vi "Journal.vi"(11 "Journal Queue":refnum<queue>) -> ()   [LabVIEW 2013, in "main.lvlib"]
uses:
  main.lvlib
  Components/Dependencies.llb/amc_Message Queue.ctl
  Components/Dependencies.llb/amc_Message.ctl
  <vilib>/FTP/util/Keyed Array.ctl
  Controls/Enum Variables.ctl
  Controls/Reference AE Control.ctl
  Components/Dependencies.llb/TLB_Dependencies.lvlib
  <vilib>/FTP/NI_FTP.lvlib
panel:
  in  "Send To PACS":bool
  in  "Stop":bool
  in  "ReportSelection":u16(ring) caption="Journal" items=["Distal Tryk", "Hudperfusionstryk", "Distal Tryk: Finger", "Arbejdstest", "Finger stimulering"]
  in  "GenerateReport":bool
  in  "Data Menu":string(tree) caption="TreeMenu"
  in  "Data Listbox":i32(listbox)=-1
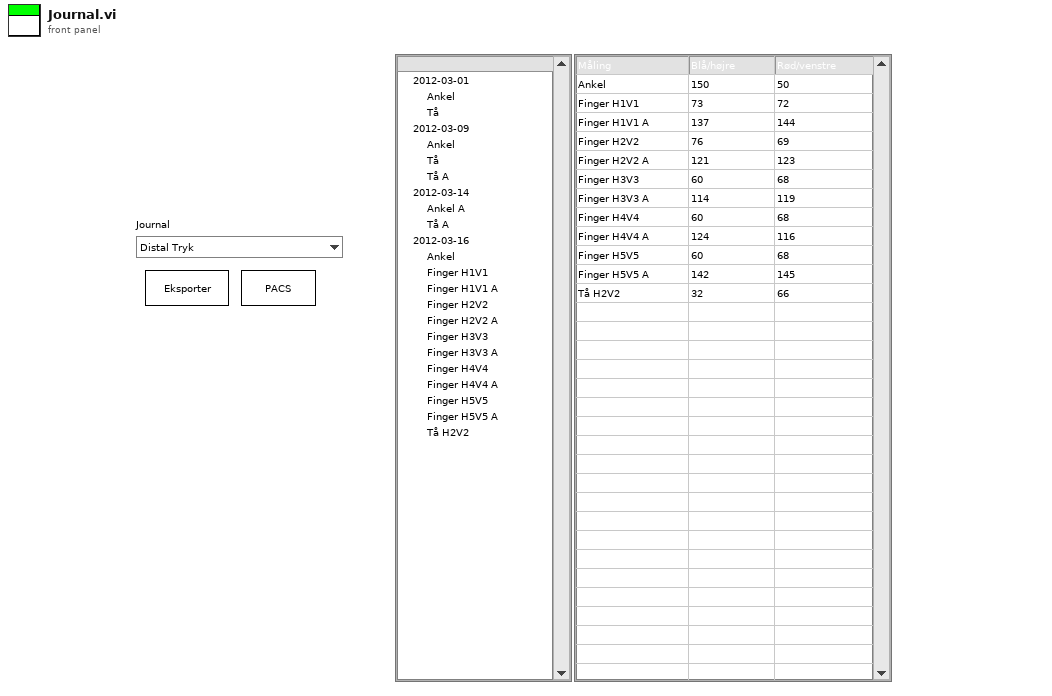
[diagram p1: front panel]
types:
  T1 = typedef "main.lvlib/TLB_Dependencies.lvlib/amc_Message Queue.ctl" = refnum<queue>
  T2 = typedef "main.lvlib/Reference AE Control.ctl" = enum16{"Initialize", "Set Menu", "Set Profile", "Set Configuration", "Set Configuration_old", "Set Configuration_new", "Set Configuration Method", "Set Acquisition", "Set Data", "Set Journal", "Get"}
  T3 = cluster{"ReportSelection":refnum<vi>, "Data Listbox":refnum<vi>, "GenerateReport":refnum<vi>, "Data Menu":refnum<vi>, "Send To PACS":refnum<vi>}
  T4 = typedef "main.lvlib/Enum Variables.ctl" = enum16{"SetAcqFilter", "GetAcqFilter", "Set Filter", "Get Filter", "Set Height", "Get Height", "Set Recorded Height", "Get Recorded Height", "Set Blue Pressure", "Get Blue Pressure", "Set Red Pressure", "Get Red Pressure", "Init", "Reset Pressure", "Set Red Cursors", "Get Red Cursors", "Set Blue Cursors", "Get Blue Cursors", "Set Language", "Get Language", "Set Active Graphs", "Get ActiveGraphs", "Set Method", "Get Method", "Set Encryption", "Get Encryption", "Set ExcelVersion", "Get ExcelVersion", "Set DICOM Avail", "Get DICOM Avail", "Set DICOM Encode", "Get DICOM Encode", "Set JournalExport", "Get JournalExport", "Set Sequence", "Get Sequence", "Set DAQ Connected", "Get DAQ Connected", "Set Current Graph", "Get Current Graph", "Set General Settings", "Get Hyphenation", "Set Arm Calc Method", "Get Arm Calc Method", "Set Dicom Tags", "Get Dicom Tags", "Set BT Serial", "Get BT Serial", "Set BT Accepted Serials", "Get BT Accepted Serials", "Get BT License", "Set BT License"}
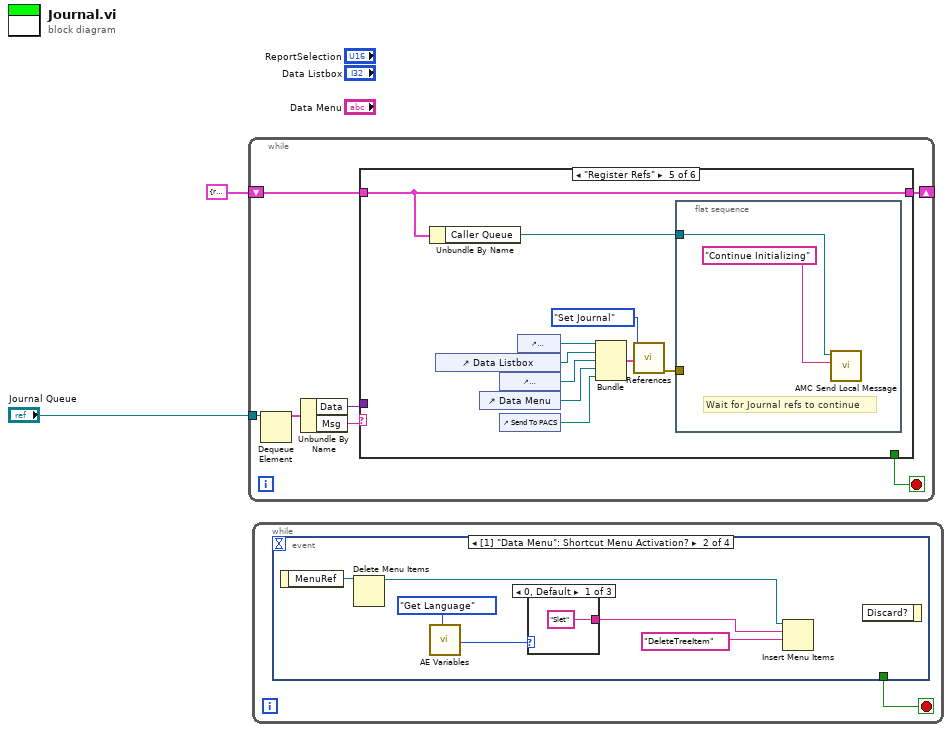
[diagram p0: block diagram]
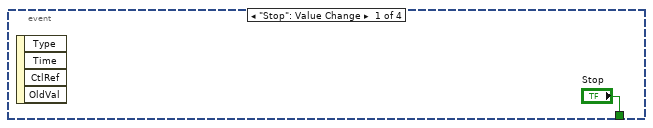
[diagram p2: hidden frame]
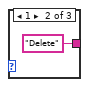
[diagram p3: hidden frame]
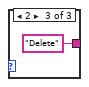
[diagram p4: hidden frame]
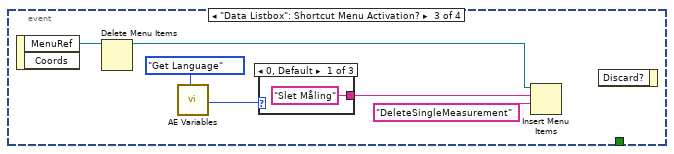
[diagram p5: hidden frame]
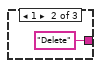
[diagram p6: hidden frame]
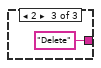
[diagram p7: hidden frame]
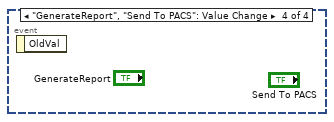
[diagram p8: hidden frame]
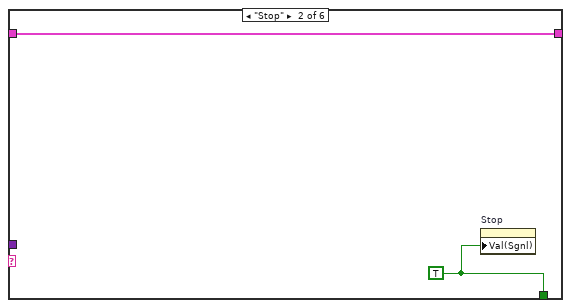
[diagram p10: hidden frame]
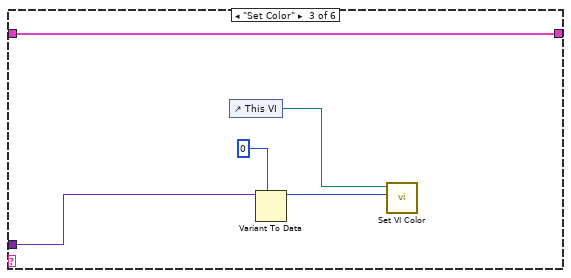
[diagram p11: hidden frame]
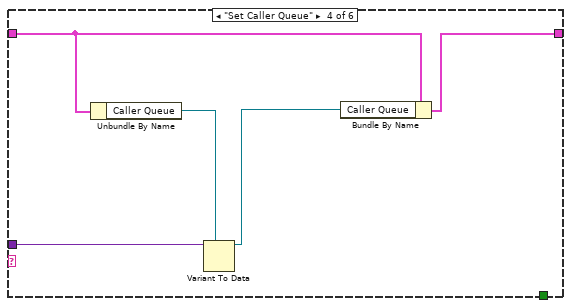
[diagram p12: hidden frame]
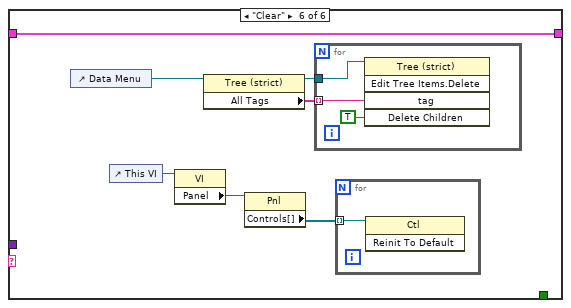
[diagram p13: hidden frame]
diagram:
  n1 = while {
    tunnel: "Journal Queue" -> [w8]
    shift-right: [w3] -> _
    shift-left: cluster{"Caller Queue":T1} {"Caller Queue"=refnum} -> [w4]
    stop <- w9 stop-if-true
    n2 = Dequeue Element(queue=w8) -> (element=w7:cluster{"Msg":string, "Data":variant})  [unwired: 2 in, 3 out]
    n3 = Unbundle By Name(w7) -> ("Data"=w5:variant, "Msg"=w6:string)
    n4 = case shown="\"Register Refs\"" w6 {
      tunnel: [_ w11 _ _ _ _] -> w9
      tunnel: w5 -> [_ _ w14 w22 _ _]
      tunnel: w4 -> [w10 w12 w13 w19 w32 w38]
      tunnel: [w10 w12 w13 w20 w32 w38] -> w3
      frame "", Default {
      }
      frame "Stop" {
        w11 = TRUE
        n5 = property on="Stop" class="Bool (strict)"("Val(Sgnl)"=w11) -> ()  [unwired: 2 in, 2 out]
      }
      frame "Set Color" {
        n6 = control-ref of="This VI"() -> (w17:refnum<vi>)
        n7 = Variant To Data(type=u32 0 ("Pane Color"), Variant=w14) -> (data=w15:u32)  [unwired: 1 in, 1 out]
        n8 = call "Set VI Color.vi"("Pane Color"=w15, "VI in"=w17) -> ()  [unwired: 10 in]
      }
      frame "Set Caller Queue" {
        n9 = Unbundle By Name(w19) -> ("Caller Queue"=w18:T1)
        n10 = Variant To Data(type=w18, Variant=w22) -> (data=w21:T1)  [unwired: 1 in, 1 out]
        n11 = Bundle By Name(cluster=w19, "Caller Queue"=w21) -> (w20:cluster{"Caller Queue":T1})
      }
      frame "Register Refs" {
        n12 = Unbundle By Name(w32) -> ("Caller Queue"=w25:T1)
        n13 = control-ref of="Data Listbox"() -> (w27:refnum<vi>)
        n14 = control-ref of="Data Menu"() -> (w29:refnum<vi>)
        n15 = control-ref of="GenerateReport"() -> (w28:refnum<vi>)
        n16 = control-ref of="Send To PACS"() -> (w24:refnum<vi>)
        n17 = control-ref of="ReportSelection"() -> (w26:refnum<vi>)
        n18 = Bundle("ReportSelection"=w26, "Data Listbox"=w27, "GenerateReport"=w28, "Data Menu"=w29, "Send To PACS"=w24) -> (w31:T3)  [unwired: 1 in]
        n19 = call "References.vi"("variant"=w31, "Reference AE Control"=Reference_AE_Control."Set Journal") -> ("error out"=w23:errorcluster)  [unwired: 8 in, 1 out]
        n20 = flat-sequence {
          tunnel: w25 -> [w34]
          tunnel: w23 -> [_]
          frame #0 {
            # "Wait for Journal refs to continue"
            n21 = call "AMC Send Local Message.vi"("Message Name"="Continue Initializing", "Message Queue in"=w34) -> ()  [unwired: 8 in, 2 out]
          }
        }
      }
      frame "Clear" {
        n22 = control-ref of="Data Menu"() -> (w36:refnum<vi>)
        n23 = control-ref of="This VI"() -> (w41:refnum<vi>)
        n24 = property class="VI"(reference=w41) -> ("Panel"=w40:refnum<vi>)  [unwired: 1 in, 2 out]
        n25 = property on="Property Node" class="Tree (strict)"(reference=w36) -> (reference out=w35:refnum<vi>, "All Tags"=w37:string[])  [unwired: 1 in, 1 out]
        n26 = property class="Pnl"(reference=w40) -> ("Controls[]"=w39:refnum<vi>[])  [unwired: 1 in, 2 out]
        n27 = for {
          tunnel: w37 -> [w44] mode=indexing
          tunnel: w35 -> [w42]
          n28 = invoke on="Invoke Node" class="Tree (strict)" method="Edit Tree Items.Delete"(reference=w42, "tag"=w44, "Delete Children"=TRUE ("Delete Children?")) -> ()  [unwired: 2 in, 5 out]
        }
        n29 = for {
          tunnel: w39 -> [w45] mode=indexing
          n30 = invoke class="Ctl" method="Reinit To Default"(reference=w45) -> ()  [unwired: 2 in, 3 out]
        }
      }
    }
  }
  n31 = while {
    stop <- w46 stop-if-true
    n32 = event shown="[1] \"Data Menu\": Shortcut Menu Activation?" {
      selector: _ -> [_ _ _ _]
      dyn-events: _ -> [_ _ _ _]
      timeout: _ -> [_ _ _ _]
      tunnel: ["Stop" _ _ _] -> w46
      event "Stop": Value Change {
        n33 = event-data() -> ()  [unwired: 1 in, 4 out]
      }
      event "Data Menu": Shortcut Menu Activation? {
        n34 = event-data() -> ("MenuRef"=w53:refnum<k9>)  [unwired: 1 in]
        n35 = Delete Menu Items(9:w53) -> (3:w50:refnum<k9>)  [unwired: 3 in, 1 out]
        n36 = call "AE Variables.vi"("Action"=Enum_Variables."Get Language") -> ("RingOut"=w48:u16)  [unwired: 11 in, 7 out]
        n37 = case shown="0, Default" w48 {
          tunnel: ["Slet" "Delete" "Delete"] -> w52
          frame 0, Default {
          }
          frame 1 {
          }
          frame 2 {
          }
        }
        n38 = Insert Menu Items(7:"DeleteTreeItem", 8:w52, 9:w50) -> ()  [unwired: 3 in, 3 out]
        n39 = event-data() -> ()  [unwired: 2 in, 1 out]
      }
      event "Data Listbox": Shortcut Menu Activation? {
        n40 = event-data() -> ("MenuRef"=w59:refnum<k9>)  [unwired: 1 in, 1 out]
        n41 = Delete Menu Items(9:w59) -> (3:w60:refnum<k9>)  [unwired: 3 in, 1 out]
        n42 = call "AE Variables.vi"("Action"=Enum_Variables."Get Language") -> ("RingOut"=w57:u16)  [unwired: 11 in, 7 out]
        n43 = case shown="0, Default" w57 {
          tunnel: ["Slet Måling" "Delete" "Delete"] -> w62
          frame 0, Default {
          }
          frame 1 {
          }
          frame 2 {
          }
        }
        n44 = Insert Menu Items(7:"DeleteSingleMeasurement", 8:w62, 9:w60) -> ()  [unwired: 3 in, 3 out]
        n45 = event-data() -> ()  [unwired: 2 in, 1 out]
      }
      event "GenerateReport", "Send To PACS": Value Change {
        n46 = event-data() -> ()  [unwired: 1 in, 1 out]
      }
    }
  }
